vi "Exit.vi"(8 "error in (no error)":errorcluster, 11 "Old State":refnum<class "Work.lvclass">) -> (0 "error out":errorcluster, 3 "New State":refnum<class "Work.lvclass">)   [LabVIEW 2024, in "Chef State.lvlib" / "Work.lvclass"]
doc: "This is an abstract method. Override this method to define the behavior when you leave the state."
uses:
  Work.lvclass
  Work.lvclass/Work.ctl
  Chef State/Chef State.lvclass
  <vilib>/ActorFramework/Actor/Actor.lvclass
  Chef UI Logic/Chef UI Logic Messages/Update Log Msg/Update Log Msg.lvclass
  C:/Users/burakkorkmaz/Desktop/PROJE/actor-state-machine/Chef State/Chef State/Chef State.lvclass
  C:/Program Files/National Instruments/LabVIEW 2024/vi.lib/NI/Actors/State Actor/State Actor/State Actor.lvclass
  C:/Program Files/National Instruments/LabVIEW 2024/vi.lib/ActorFramework/Actor/Actor.lvclass
  C:/Users/burakkorkmaz/Desktop/PROJE/actor-state-machine/Chef State/Work/Work.lvclass
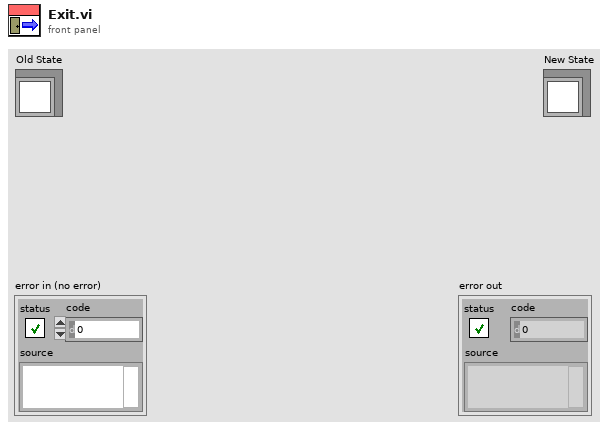
[diagram p1: front panel]
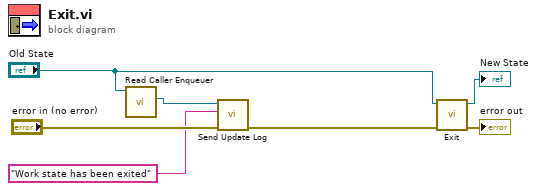
[diagram p0: block diagram]
diagram:
  n1 = call <vilib>:"Read Caller Enqueuer.vi"("Actor"="Old State") -> ("Caller Enqueuer"=w3:refnum<class "Message Enqueuer.lvclass">)  [unwired: 10 in]
  n2 = call "Send Update Log.vi"("error in (no error)"="error in (no error)", "Log"="Work state has been exited", "Message Enqueuer"=w3) -> ("error out"=w4:errorcluster)  [unwired: 7 in, 1 out]
  n3 = call-parent "Exit.vi"("error in (no error)"=w4, "Old State"="Old State") -> ("error out"=→"error out":errorcluster, "New State"=→"New State":refnum<class "Work.lvclass">)  [unwired: 8 in]
